vi "Run.vi"(8 "error in (no error)":errorcluster, 11 "Socket in":refnum<class "Socket.lvclass">) -> (0 "error out":errorcluster, 3 "Socket out":refnum<class "Socket.lvclass">)   [LabVIEW 2018, in "Socket.lvclass"]
uses:
  Socket.lvclass
  Socket.lvclass/Socket.ctl
  State Machine/CM_State Machine.lvclass
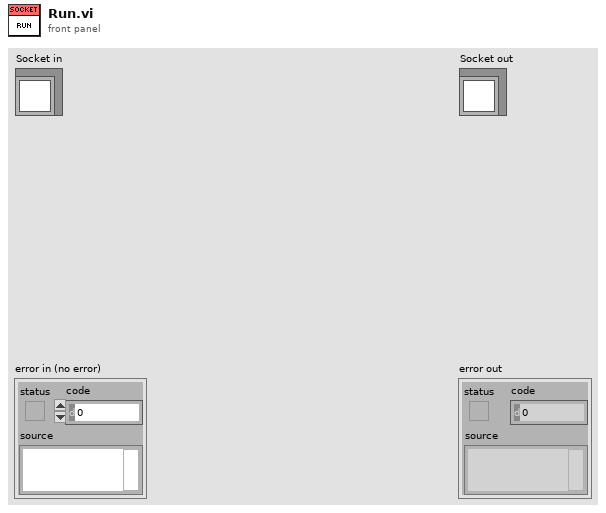
[diagram p1: front panel]
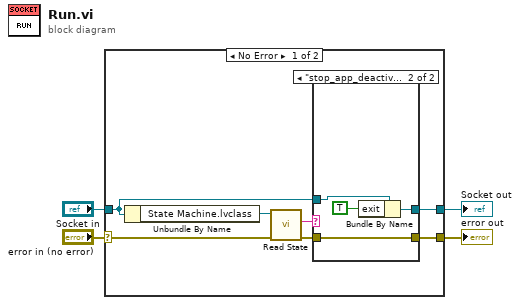
[diagram p0: block diagram]
diagram:
  n1 = case shown="No Error" "error in (no error)" {
    selector: "error in (no error)" -> [w10 w19]
    tunnel: [w7 w19] -> w3
    tunnel: [w5 w18] -> w1
    tunnel: "Socket in" -> [w6 w18]
    frame No Error {
      n2 = Unbundle By Name(w6) -> ("State Machine.lvclass"=w11:refnum<class "CM_State Machine.lvclass">)
      n3 = call-dynamic "Read State.vi"("error in (no error)"=w10, "State Machine in"=w11) -> ("error out"=w8:errorcluster, "State"=w9:string)  [unwired: 7 in, 1 out]
      n4 = case shown="\"stop_app_deactivated\"" w9 {
        tunnel: w8 -> [w12 w17]
        tunnel: [w12 w17] -> w7
        tunnel: w6 -> [w13 w16]
        tunnel: [w13 w14] -> w5
        frame "False", Default {
        }
        frame "stop_app_deactivated" {
          n5 = Bundle By Name(cluster=w16, "exit"=TRUE) -> (w14:refnum<class "Socket.lvclass">)
        }
      }
    }
    frame Error {
    }
  }
  "error out" <- w3
  "Socket out" <- w1
